vi "Adjust Dashboard Window.vi"(6 "Sizing Refnums":T1, 9 "Size Constraints":cluster{"min tab width":i32, "w/h":dbl}, 10 "VI":refnum<vi>, 11 "Notifier in":refnum<notifier>) -> ()   [LabVIEW 2014]
uses:
  <vilib>/Utility/miscctls.llb/LVRectTypeDef.ctl
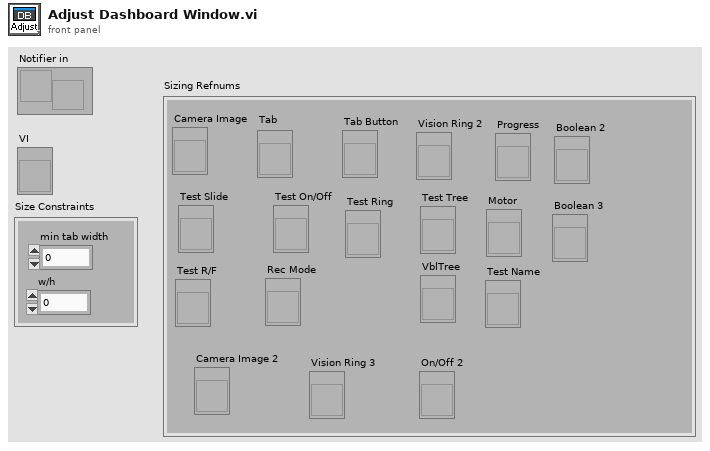
[diagram p1: front panel]
types:
  T1 = cluster{"Camera Image":refnum<vi>, "Tab":refnum<vi>, "Tab Button":refnum<vi>, "Vision Ring 2":refnum<vi>, "Rec Mode":refnum<vi>, "Test Slide":refnum<vi>, "Test On/Off":refnum<vi>, "Test Ring":refnum<vi>, "Test R/F":refnum<vi>, "Test Name":refnum<vi>, "Motor":refnum<vi>, "Progress":refnum<vi>, "Test Tree":refnum<vi>, "VblTree":refnum<vi>, "Boolean 2":refnum<vi>, "Boolean 3":refnum<vi>, "Camera Image 2":refnum<vi>, "Vision Ring 3":refnum<vi>, "On/Off 2":refnum<vi>}
  T2 = typedef "LVRectTypeDef.ctl" = cluster{"Left":i16, "Top":i16, "Right":i16, "Bottom":i16}
  T3 = typedef "LVPointTypeDef.ctl" = cluster{"Horizontal":i16, "Vertical":i16}
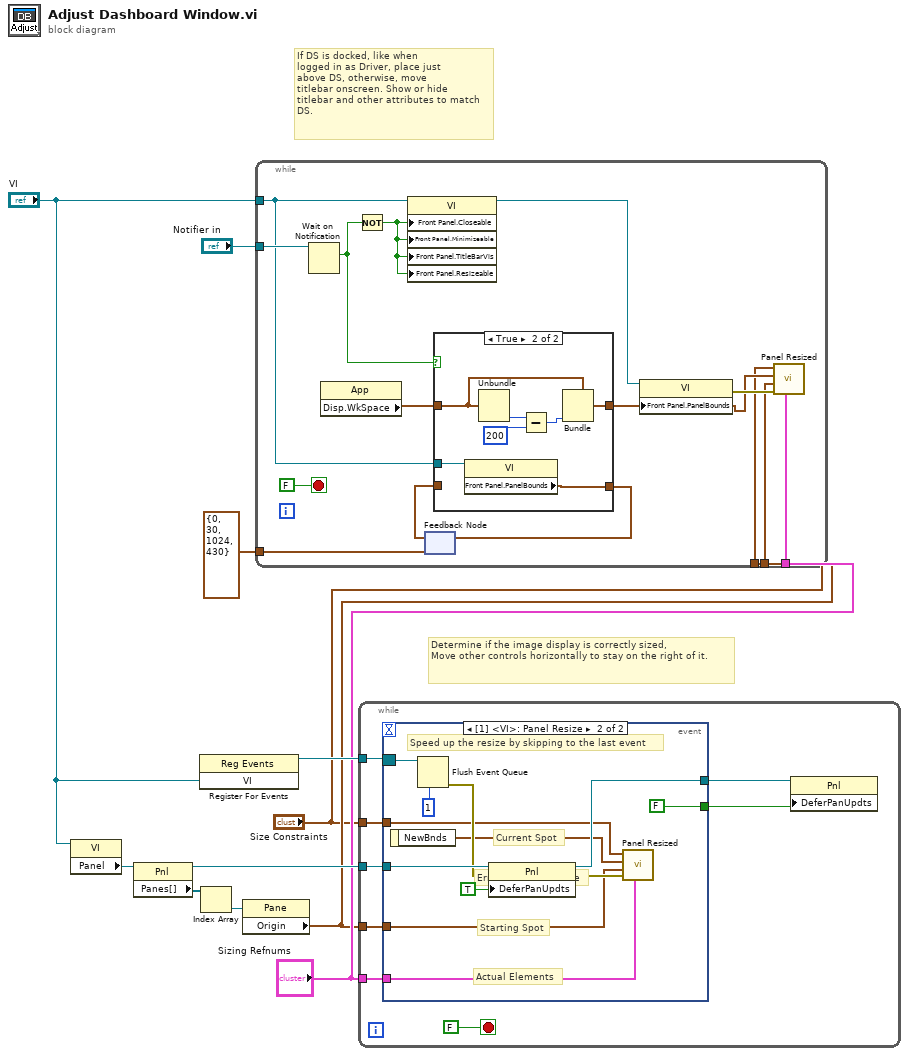
[diagram p0: block diagram]
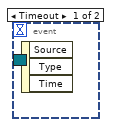
[diagram p2: hidden frame]
diagram:
  # "Determine if the image display is correctly sized,\nMove other controls horizontally to stay on the right of it."
  # "If DS is docked, like when\nlogged in as Driver, place just\nabove DS, otherwise, move\ntitlebar onscreen. Show or hide\ntitlebar and other attributes to match\nDS."
  n1 = property class="VI"(reference="VI") -> ("Panel"=w8:refnum<vi>)  [unwired: 1 in, 2 out]
  n2 = property class="Pnl"(reference=w8) -> (reference out=w5:refnum<vi>, "Panes[]"=w7:refnum<vi>[])  [unwired: 1 in, 1 out]
  n3 = register-events("VI") -> (reference out=w10:refnum<event-registration>)  [unwired: 2 in, 1 out]
  n4 = Index Array(array=w7) -> (element=w6:refnum<vi>)  [unwired: 1 in]
  n5 = property class="Pane"(reference=w6) -> ("Origin"=w3:T3)  [unwired: 1 in, 2 out]
  n6 = while {
    tunnel: "Notifier in" -> [w25]
    tunnel: "VI" -> [w16]
    tunnel: "Sizing Refnums" -> [w21]
    tunnel: w3 -> [w20]
    tunnel: "Size Constraints" -> [w18]
    tunnel: T2 {"Left"=0, "Top"=30, "Right"=1024, "Bottom"=430} ("Front Panel.PanelBounds") -> [w13]
    stop <- FALSE stop-if-true
    n7 = Wait on Notification(notifier=w25) -> (notification=w17:bool)  [unwired: 3 in, 3 out]
    n8 = property class="App"() -> ("Disp.WkSpace"=w24:T2)  [unwired: 2 in, 2 out]
    n9 = Not(x=w17) -> (.not. x?=w12:bool)
    n10 = property class="VI"(reference=w16, "Front Panel.Closeable"=w12, "Front Panel.Minimizeable"=w12, "Front Panel.TitleBarVis"=w12, "Front Panel.Resizeable"=w12) -> (reference out=w23:refnum<vi>)  [unwired: 1 in, 1 out]
    n11 = feedback #1(w13) -> (w14:T2)
    n12 = case shown="True" w17 {
      tunnel: w24 -> [_ w30]
      tunnel: [w27 w31] -> w19
      tunnel: w16 -> [_ w29]
      tunnel: [w27 w28] -> w15
      tunnel: w14 -> [w27 _]
      frame False {
      }
      frame True {
        n13 = property class="VI"(reference=w29) -> ("Front Panel.PanelBounds"=w28:T2)  [unwired: 1 in, 2 out]
        n14 = Unbundle(w30) -> ("Bottom"=w34:i16)  [unwired: 3 out]
        n15 = Subtract(x=w34, y=200) -> (x-y=w32:i32)
        n16 = Bundle(cluster=w30, "Bottom"=w32) -> (w31:T2)  [unwired: 3 out]
      }
    }
    n17 = feedback-in #1(w15) -> ()
    n18 = property class="VI"(reference=w23, "Front Panel.PanelBounds"=w19) -> (error out=w22:errorcluster)  [unwired: 1 in, 1 out]
    n19 = call "Panel Resized.vi"("Sizing Refnums"=w21, "error in (no error)"=w22, "Origin"=w20, "NewBnds"=w19, "Size Constraints"=w18) -> ()  [unwired: 6 in, 1 out]
  }
  n20 = while {
    tunnel: w10 -> [w41]
    tunnel: "Sizing Refnums" -> [w40]
    tunnel: "Size Constraints" -> [w39]
    tunnel: w3 -> [w38]
    tunnel: w5 -> [w37]
    stop <- FALSE stop-if-true
    n21 = event shown="[1] <VI>: Panel Resize" {
      selector: w41 -> [_ w51]
      dyn-events: _ -> [_ _]
      timeout: _ -> [_ _]
      tunnel: w40 -> [_ w43]
      tunnel: w39 -> [_ w46]
      tunnel: w38 -> [_ w44]
      tunnel: w37 -> [_ w54]
      tunnel: [_ FALSE ("Defer Panel Updates")] -> w36
      tunnel: [_ w48] -> w35
      event Timeout {
        n22 = event-data() -> ()  [unwired: 1 in, 3 out]
      }
      event Panel Resize {
        # "Error for Panel Resize"
        # "Actual Elements"
        # "Current Spot"
        # "Starting Spot"
        # "Speed up the resize by skipping to the last event"
        n23 = event-data() -> ("NewBnds"=w45:T2)  [unwired: 1 in]
        n24 = Flush Event Queue(0:w51, 5:1 ("keep most recent")) -> (11:w49:errorcluster)  [unwired: 4 in, 2 out]
        n25 = property class="Pnl"(reference=w54, error in=w49, "DeferPanUpdts"=TRUE ("Defer Panel Updates")) -> (reference out=w48:refnum<vi>, error out=w47:errorcluster)
        n26 = call "Panel Resized.vi"("Sizing Refnums"=w43, "error in (no error)"=w47, "Origin"=w44, "NewBnds"=w45, "Size Constraints"=w46) -> ()  [unwired: 6 in, 1 out]
      }
    }
    n27 = property class="Pnl"(reference=w35, "DeferPanUpdts"=w36) -> ()  [unwired: 1 in, 2 out]
  }
